vi "Swap Topology.vi"(8 "error in (no error)":errorcluster, 9 "reset device (boolean value)":bool=TRUE, 10 "Topology":string, 11 "SLSC Switch in":refnum<class "SLSC Switch.lvclass">) -> (0 "error out":errorcluster, 3 "SLSC Switch out":refnum<class "SLSC Switch.lvclass">)   [LabVIEW 2015, in "SLSC Switch.lvlib" / "SLSC Switch.lvclass"]
uses:
  SLSC Switch.lvclass
  SLSC Switch.lvclass/SLSC Switch.ctl
  slscsl/slscsl.lvclass
  SLSC Session/SLSC Session.lvclass
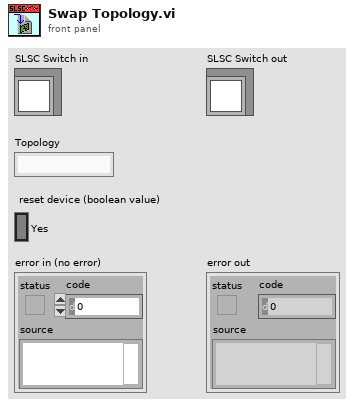
[diagram p1: front panel]
types:
  T1 = typedef "SLSC Switch.lvlib/SLSC Session.lvclass/Session Handle.ctl" = refnum<data-value>
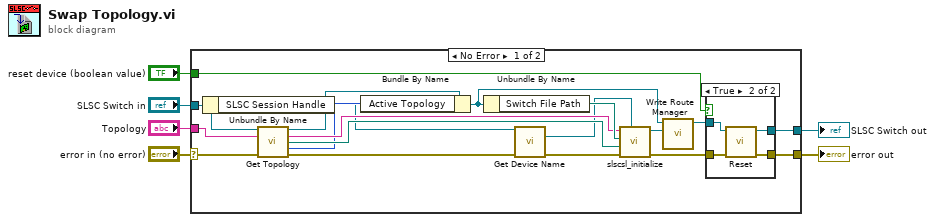
[diagram p0: block diagram]
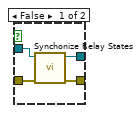
[diagram p2: hidden frame]
diagram:
  n1 = case shown="No Error" "error in (no error)" {
    selector: "error in (no error)" -> [w24 w35]
    tunnel: [w21 w35] -> w5
    tunnel: [w22 w34] -> w3
    tunnel: "SLSC Switch in" -> [w25 w34]
    tunnel: "reset device (boolean value)" -> [w18 _]
    tunnel: "Topology" -> [w23 _]
    frame No Error {
      n2 = Unbundle By Name(w25) -> ("SLSC Session Handle"=w10:T1)
      n3 = call "Get Topology.vi"("SLSC Switch in"=w25, "Topology Name In"=w23, "error in (no error)"=w24) -> ("SLSC Switch out"=w13:refnum<class "SLSC Switch.lvclass">, "Topology Name Out"=w14:string, "Topology File Path out"=w15:path, "Active Index"=w12:i32, "error out"=w8:errorcluster)  [unwired: 8 in]
      n4 = Bundle By Name(cluster=w13, "Active Topology"=w12) -> (w11:refnum<class "SLSC Switch.lvclass">)
      n5 = Unbundle By Name(w11) -> ("Switch File Path"=w16:path)
      n6 = call "Get Device Name.vi"("Session Handle in"=w10, "error in (no error)"=w8) -> ("device"=w9:refnum<k21>, "error out"=w7:errorcluster)  [unwired: 11 in, 1 out]
      n7 = call "slscsl_initialize.vi"("deviceIdentifier"=w9, "error in (no error)"=w7, "top file path"=w15, "shw file path"=w16, "topologyName"=w14) -> ("error out"=w20:errorcluster, "slscsl out"=w17:refnum<class "slscsl.lvclass">)  [unwired: 5 in]
      n8 = call "Write Route Manager.vi"("Route Manager.lvclass"=w17, "SLSC Switch in"=w11) -> ("SLSC Switch out"=w19:refnum<class "SLSC Switch.lvclass">)  [unwired: 9 in]
      n9 = case shown="True" w18 {
        tunnel: w20 -> [w29 w32]
        tunnel: [w28 w31] -> w21
        tunnel: [w27 w30] -> w22
        tunnel: w19 -> [w26 w33]
        frame False {
          n10 = call "Synchonize Relay States.vi"("error in (no error)"=w29, "SLSC Switch in"=w26) -> ("error out"=w28:errorcluster, "SLSC Switch out"=w27:refnum<class "SLSC Switch.lvclass">)  [unwired: 8 in]
        }
        frame True {
          n11 = call "Reset.vi"("error in (no error)"=w32, "SLSC Switch in"=w33) -> ("error out"=w31:errorcluster, "SLSC Switch out"=w30:refnum<class "SLSC Switch.lvclass">)  [unwired: 8 in]
        }
      }
    }
    frame Error {
    }
  }
  "error out" <- w5
  "SLSC Switch out" <- w3
